vi "Write Textual.vi"(8 "error in (no error)":errorcluster, 10 "Textual":bool, 11 "TCP Listener in":refnum<class "TCP Listener.lvclass">) -> (0 "error out":errorcluster, 3 "TCP Listener out":refnum<class "TCP Listener.lvclass">)   [LabVIEW 2020, in "TALOS.lvlib" / "TCP Listener.lvlib" / "TCP Listener.lvclass"]
uses:
  TCP Listener.lvclass
  TCP Listener.lvclass/TCP Listener.ctl
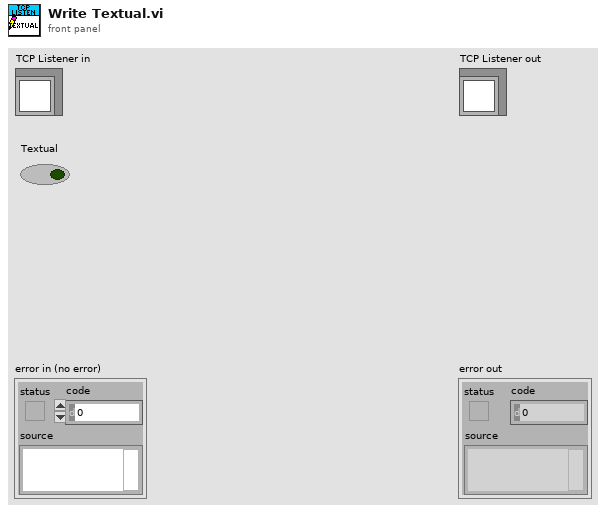
[diagram p1: front panel]
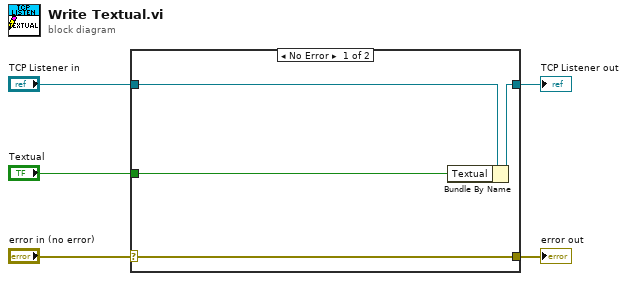
[diagram p0: block diagram]
diagram:
  n1 = case shown="No Error" "error in (no error)" {
    selector: "error in (no error)" -> [w9 w10]
    tunnel: [w9 w10] -> w4
    tunnel: [w7 w11] -> w2
    tunnel: "TCP Listener in" -> [w8 w11]
    tunnel: "Textual" -> [w6 _]
    frame No Error {
      n2 = Bundle By Name(cluster=w8, "Textual"=w6) -> (w7:refnum<class "TCP Listener.lvclass">)
    }
    frame Error {
    }
  }
  "error out" <- w4
  "TCP Listener out" <- w2
